vi "DAQ Encoder_Vibration_Microphone.vi"() -> ()   [LabVIEW 2021]
doc: "This example demonstrates how to continuously acquire buffered voltage measurements using a DAQmx device.\n\nFor instructions on how to connect your signals to the DAQ device, refer to your device documentation."
uses:
  <vilib>/Utility/error.llb/DialogType.ctl
  <vilib>/DAQmx/read.llb/DAQmx Read (Counter 1D DBL 1Chan NSamp).vi
  <vilib>/DAQmx/read.llb/DAQmx Read (Analog 1D Wfm NChan NSamp).vi
  <vilib>/DAQmx/create/channels.llb/DAQmx Create Channel (AI-Acceleration-Accelerometer).vi
  <vilib>/DAQmx/create/channels.llb/DAQmx Create Channel (AI-Sound Pressure-Microphone).vi
  <vilib>/DAQmx/configure/timing.llb/DAQmx Timing (Sample Clock).vi
  <vilib>/DAQmx/create/channels.llb/DAQmx Create Channel (CI-Position-Angular Encoder).vi
  <vilib>/DAQmx/miscellaneous.llb/DAQmx Fill In Error Info.vi
  <resource>/objmgr/daqmx.rc
panel:
  in  "File Path":path
  in  "Encoder Channel":tag="cDAQ1Mod2/ctr0"
  in  "Microphone channels":tag="cDAQ1Mod1/ai0"
  in  "Vibration channels":tag="cDAQ1Mod1/ai1:2"
  out "RPM":dbl
  out "Time per Loop":i32
  out "Microphone":waveform(dbl)[](graph)
  in  "Stop":bool
  in  "Number of Samples":i32=100
  in  "Sample Rate":dbl=1000.0
  out "Vib2":waveform(dbl)[](graph)
  out "Vib1":waveform(dbl)[](graph)
  # "Encoder Settings"
  # "Vibration  X"
  # "AI Channel Settings"
  # "Vibration Y"
  # "Operations"
  # "Microphone"
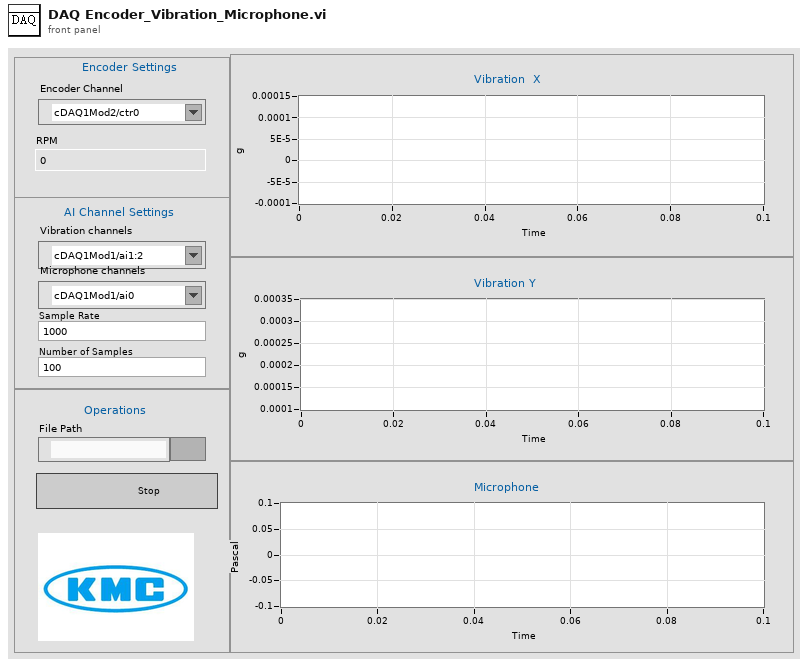
[diagram p1: front panel]
types:
  T1 = enum16{"open", "replace", "create", "open or create", "replace or create", "replace or create with confirmation"}
  T2 = typedef "DialogType.ctl" = u16
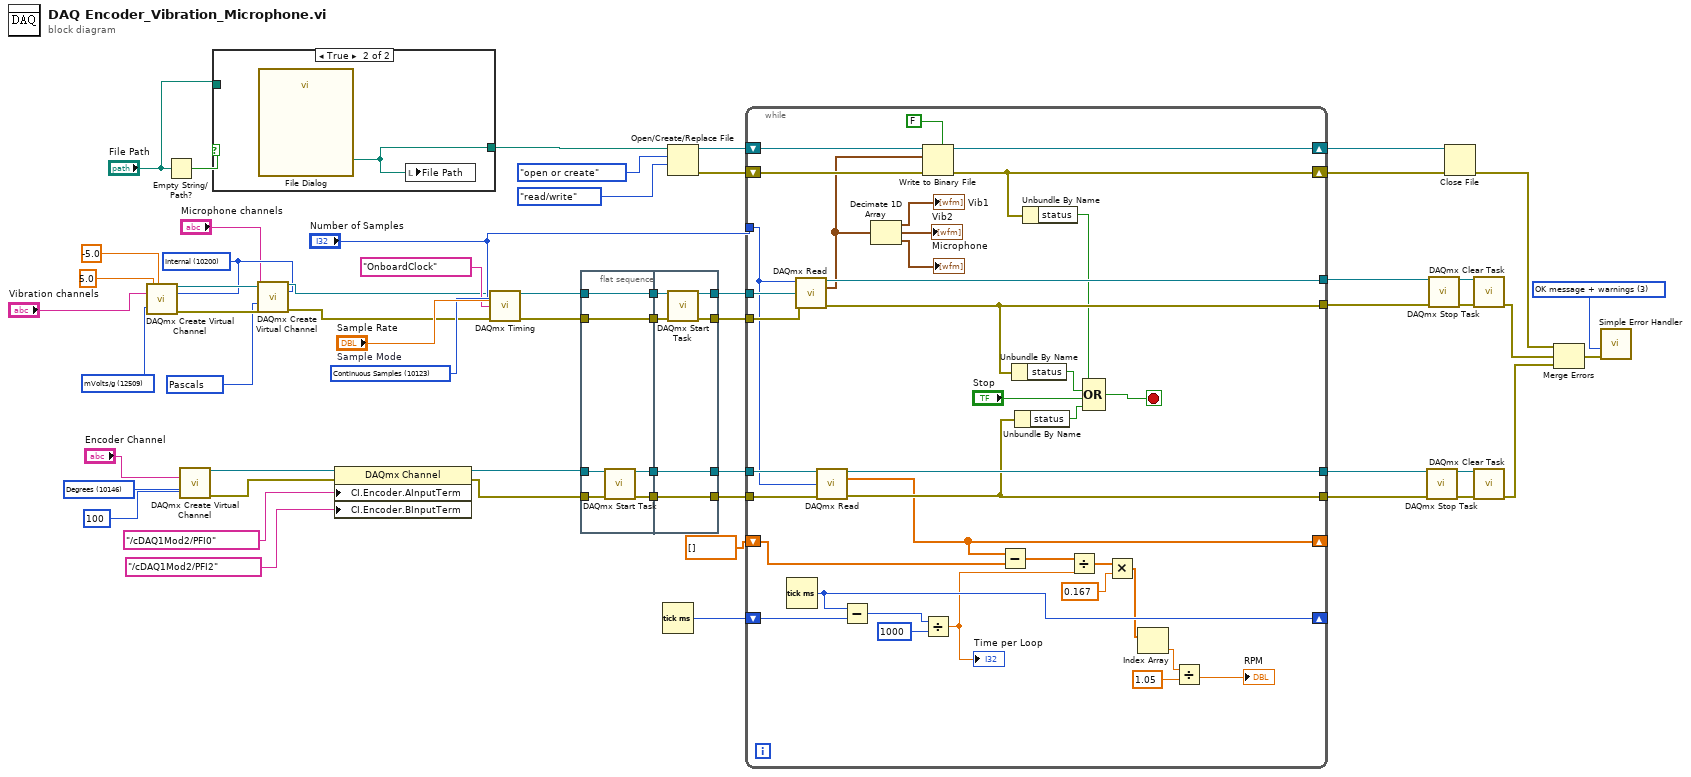
[diagram p0: block diagram]
diagram:
  w7 = 10081 items=["Pascals"=10081, "From Custom Scale"=10065] ("units")
  w8 = 12509 items=["mVolts/g"=12509, "Volts/g"=12510] ("sensitivity units")
  w9 = 10200 items=["Internal"=10200, "External"=10167, "None"=10230] ("current excitation source")
  w22 = 10146 items=["Degrees"=10146, "Radians"=10273, "Ticks"=10304, "From Custom Scale"=10065] ("units")
  w55 = T2 3 items=["no dialog", "OK message", "continue or stop message", "OK message + warnings", "continue/stop + warnings"] ("type of dialog (OK msg:1)")
  w38 = 10123 items=["Finite Samples"=10178, "Continuous Samples"=10123, "Hardware Timed Single Point"=12522]  # Sample Mode
  n1 = call-poly <vilib>:"DAQmx Create Virtual Channel.vi"("maximum value"=5.0, "minimum value"=-5.0, "physical channels"="Vibration channels", "current excitation source"=w9, "sensitivity units"=w8) -> ("task out"=w14:refnum<k21>, "error out"=w13:errorcluster)  [unwired: 9 in]
  n2 = Empty String/Path?(string/path="File Path") -> (empty?=w3:bool)
  n3 = call-poly <vilib>:"DAQmx Create Virtual Channel.vi"("counter"="Encoder Channel", "units"=w22, "pulses per revolution"=u32 100) -> ("task out"=w52:refnum<k21>, "error out"=w50:errorcluster)  [unwired: 11 in]
  n4 = case shown="True" w3 {
    tunnel: "File Path" -> [w59 _]
    tunnel: [w59 w60] -> w1
    frame False {
    }
    frame True {
      n5 = call "File Dialog"() -> ("selected path"=w60:path)  [unwired: 12 in, 3 out]
      n6 = local write "File Path"(w60) -> ()
    }
  }
  n7 = call-poly <vilib>:"DAQmx Create Virtual Channel.vi"("task in"=w14, "physical channels"="Microphone channels", "current excitation source"=w9, "units"=w7, "error in"=w13) -> ("task out"=w12:refnum<k21>, "error out"=w11:errorcluster)  [unwired: 9 in]
  n8 = property class="DAQmx Channel"(reference=w52, error in=w50, "CI.Encoder.AInputTerm"=tag "/cDAQ1Mod2/PFI0" ("A Input Terminal"), "CI.Encoder.BInputTerm"=tag "/cDAQ1Mod2/PFI2" ("B Input Terminal")) -> (reference out=w16:refnum<k21>, error out=w15:errorcluster)
  n9 = call-poly <vilib>:"DAQmx Timing.vi"("task/channels in"=w12, "sample mode"=w38, "samples per channel"="Number of Samples", "rate"="Sample Rate", "source"=tag "OnboardClock" ("AI Sample Clock Source"), "error in"=w11) -> ("task out"=w31:refnum<k21>, "error out"=w29:errorcluster)  [unwired: 8 in]
  n10 = flat-sequence {
    tunnel: [w66] -> w36
    tunnel: [w65] -> w35
    tunnel: [w64] -> w32
    tunnel: w31 -> [w64]
    tunnel: w29 -> [w63]
    tunnel: [w63] -> w30
    tunnel: w16 -> [w62]
    tunnel: w15 -> [w61]
    tunnel: [w71] -> w45
    tunnel: [w72] -> w46
    tunnel: w36 -> [w72]
    tunnel: w35 -> [w71]
    tunnel: [w70] -> w34
    tunnel: [w69] -> w33
    tunnel: w32 -> [w68]
    tunnel: w30 -> [w67]
    frame #0 {
      n11 = call <vilib>:"DAQmx Start Task.vi"("task/channels in"=w62, "error in"=w61) -> ("task out"=w66:refnum<k21>, "error out"=w65:errorcluster)  [unwired: 12 in]
    }
    frame #1 {
      n12 = call <vilib>:"DAQmx Start Task.vi"("task/channels in"=w68, "error in"=w67) -> ("task out"=w70:refnum<k21>, "error out"=w69:errorcluster)  [unwired: 12 in]
    }
  }
  n13 = Tick Count (ms)() -> (millisecond timer value=w54:u32)
  n14 = Open/Create/Replace File(file path (use dialog)=w1, operation (0:open)=T1."open or create", access (0:read/write)=enum16{"read/write", "read-only", "write-only"}."read/write") -> (refnum out=w26:refnum<file>, error out=w25:errorcluster)  [unwired: 3 in, 1 out]
  n15 = while {
    tunnel: w34 -> [w109]
    tunnel: w33 -> [w108]
    tunnel: [w107] -> w58
    tunnel: [w106] -> w53
    tunnel: "Number of Samples" -> [w97]
    shift-right: [w89] -> _
    shift-left: w54 -> [w105]
    tunnel: w46 -> [w104]
    tunnel: w45 -> [w103]
    tunnel: [w102] -> w44
    tunnel: [w101] -> w43
    shift-right: [w94] -> w24
    shift-left: w26 -> [w96]
    shift-right: [w78] -> w23
    shift-left: w25 -> [w95]
    shift-right: [w92] -> _
    shift-left: dbl[] [] ("data") -> [w91]
    stop <- w83 stop-if-true
    n16 = Tick Count (ms)() -> (millisecond timer value=w89:u32)
    n17 = call-poly <vilib>:"DAQmx Read.vi"("task/channels in"=w109, "number of samples per channel"=w97, "error in"=w108) -> ("task out"=w107:refnum<k21>, "data"=w82:waveform(dbl)[], "error out"=w106:errorcluster)  [unwired: 10 in]
    n18 = call-poly <vilib>:"DAQmx Read.vi"("task/channels in"=w104, "number of samples per channel"=w97, "error in"=w103) -> ("task out"=w102:refnum<k21>, "data"=w92:dbl[], "error out"=w101:errorcluster)  [unwired: 10 in]
    n19 = Subtract(x=w89, y=w105) -> (x-y=w88:u32)
    n20 = Decimate 1D Array(w82) -> (→"Vib1":waveform(dbl)[], →"Vib2":waveform(dbl)[], →"Microphone":waveform(dbl)[])
    n21 = Write to Binary File(file (use dialog)=w96, data=w82, error in=w95, 5:FALSE ("prepend array or string size? (T)")) -> (refnum out=w94:refnum<file>, error out=w78:errorcluster)  [unwired: 2 in, 1 out]
    n22 = Divide(x=w88, y=u32 1000) -> (x/y=w86:dbl)
    "Time per Loop" <- w86
    n23 = Subtract(x=w92, y=w91) -> (x-y=w90:dbl[])
    n24 = Unbundle By Name(w106) -> ("status"=w100:bool)
    n25 = Unbundle By Name(w101) -> ("status"=w98:bool)
    n26 = Unbundle By Name(w78) -> ("status"=w77:bool)
    n27 = Divide(x=w90, y=w86) -> (x/y=w85:dbl[])
    n28 = Compound Arithmetic op=OR(w77, w100, "Stop", w98) -> (w83:bool)
    n29 = Multiply(x=w85, y=0.167) -> (x*y=w76:dbl[])
    n30 = Index Array(array=w76) -> (element=w75:dbl)  [unwired: 1 in]
    n31 = Divide(x=w75, y=1.05) -> (x/y=→"RPM":dbl)
  }
  n32 = call <vilib>:"DAQmx Stop Task.vi"("task/channels in"=w44, "error in"=w43) -> ("task out"=w47:refnum<k21>, "error out"=w48:errorcluster)  [unwired: 12 in]
  n33 = call <vilib>:"DAQmx Stop Task.vi"("task/channels in"=w58, "error in"=w53) -> ("task out"=w56:refnum<k21>, "error out"=w57:errorcluster)  [unwired: 12 in]
  n34 = Close File(refnum=w24, error in=w23) -> (error out=w20:errorcluster)  [unwired: 1 out]
  n35 = call <vilib>:"DAQmx Clear Task.vi"("task in"=w56, "error in"=w57) -> ("error out"=w42:errorcluster)  [unwired: 13 in]
  n36 = call <vilib>:"DAQmx Clear Task.vi"("task in"=w47, "error in"=w48) -> ("error out"=w41:errorcluster)  [unwired: 13 in]
  n37 = Merge Errors(w20, w42, w41) -> (w40:errorcluster)
  n38 = call <vilib>:"Simple Error Handler.vi"("type of dialog (OK msg:1)"=w55, "error in (no error)"=w40) -> ()  [unwired: 3 in, 5 out]
